vi "Validate_Do.vi"(8 "error in (no error)":errorcluster, 11 "Action Interface in":refnum<class "Action Interface.lvclass">) -> (0 "error out":errorcluster, 1 "Valid?":bool, 3 "Action Interface out":refnum<class "Action Interface.lvclass">)   [LabVIEW 2020, in "ProjectBuilder.lvlib" / "Action Interface.lvclass"]
uses:
  Action Interface.lvclass
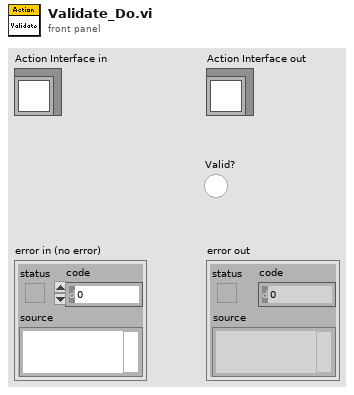
[diagram p1: front panel]
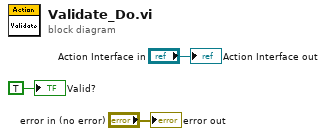
[diagram p0: block diagram]
diagram:
  "error out" <- "error in (no error)"
  "Action Interface out" <- "Action Interface in"
  "Valid?" <- TRUE
